vi "mlProject_testNetwork.vi"() -> ()   [LabVIEW 2016]
uses:
  <vilib>/Analysis/7linalg.llb/Real Matrix Exp.vi
  <vilib>/Analysis/Matrix/Numeric/Subtract/Subtract - RM,RM.vi
  <vilib>/Analysis/NI_AALBase.lvlib
  <vilib>/Analysis/Matrix/NI_Matrix.lvlib
panel:
  out "error":i32
  out "Coefficient error":sgl[][](array[numeric])
  in  "nesterov":bool=TRUE
  in  "lambda":sgl
  in  "gamma":sgl=0.9
  in  "milliseconds to wait":u32
  out "out desired":sgl[][](array[numeric])
  in  "validate":bool
  out "Error":sgl[](graph)
  in  "eta":sgl=0.0001
  in  "stop":bool
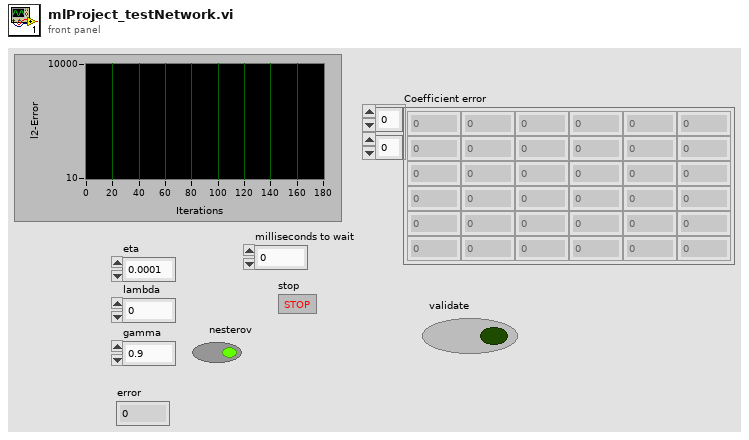
[diagram p1: front panel]
types:
  T1 = typedef "NI_Matrix.lvlib/RealMatrix.ctl" = dbl[][]
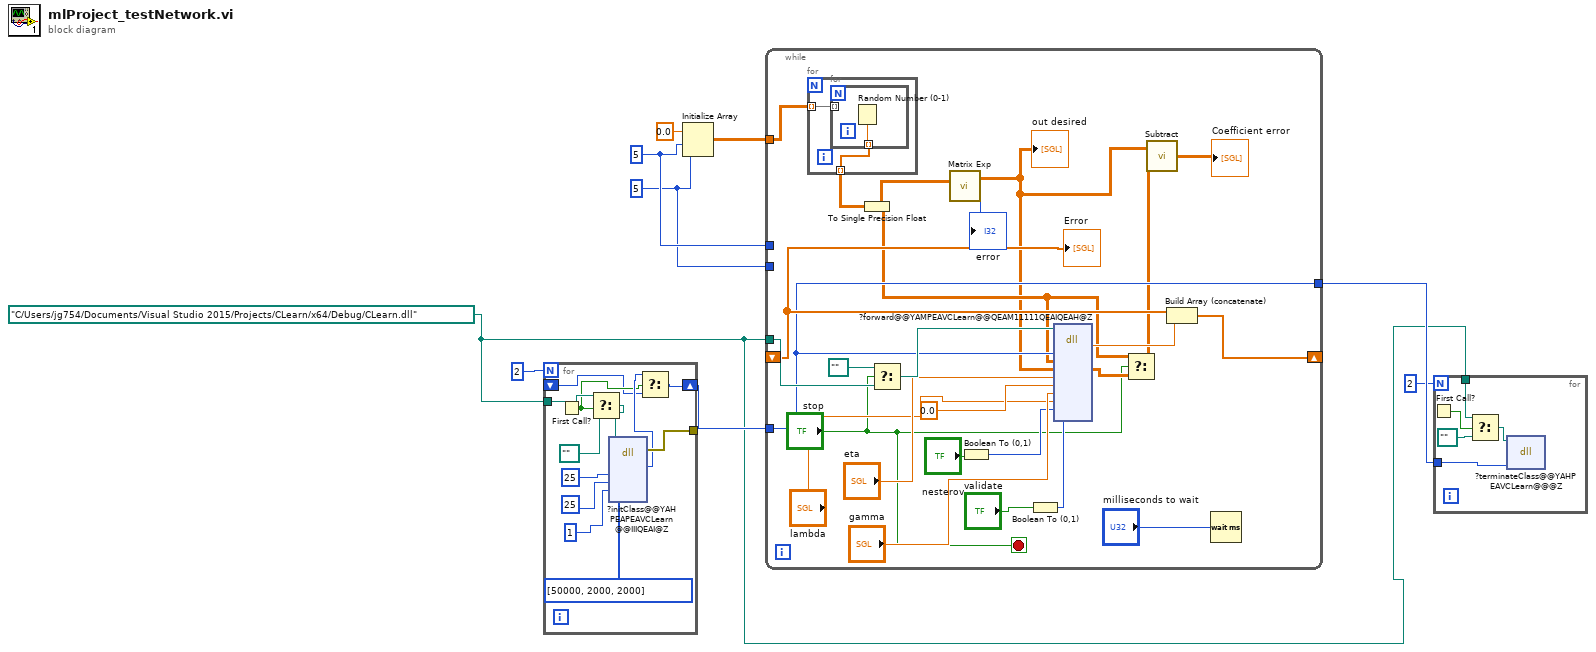
[diagram p0: block diagram]
diagram:
  w1 = 5 ("dimension size")
  w2 = 5 ("dimension size")
  w6 = path "C:/Users/jg754/Documents/Visual Studio 2015/Projects/CLearn/x64/Debug/CLearn.dll" ("path in")
  n1 = for {
    N: 2 -> [_]
    tunnel: w6 -> [w20]
    tunnel: [w21] -> _
    shift-right: [w17] -> w8
    shift-left: _ -> [w15]
    n2 = First Call?() -> (First Call?: T/F=w16:bool)
    n3 = Select(t=w20, s=w16, f=path "") -> (s? t:f=w19:path)
    n4 = dll-call lib="C:/Users/jg754/Documents/Visual Studio 2015/Projects/CLearn/x64/Debug/CLearn.dll" fn="?initClass@@YAHPEAPEAVCLearn@@IIIQEAI@Z"(path in=w19, "NIN"=u32 25, "NOUT"=u32 25, "NHIDDEN"=u32 1, "NNODES"=u32[] [50000, 2000, 2000]) -> (error out=w21:errorcluster, "ptr"=w18:i64)  [unwired: 8 in, 1 out]
    n5 = Select(t=w18, s=w16, f=w15) -> (s? t:f=w17:i64)
  }
  n6 = Initialize Array(0.0 ("element"), w2, w1) -> (w4:dbl[][])
  n7 = while {
    tunnel: w8 -> [w36]
    tunnel: w6 -> [w45]
    shift-right: [w41] -> _
    shift-left: _ -> [w40]
    tunnel: [w36] -> w7
    tunnel: w4 -> [w34]
    tunnel: w2 -> [_]
    tunnel: w1 -> [_]
    stop <- "stop" stop-if-true
    n8 = for {
      tunnel: w34 -> [w48] mode=indexing
      tunnel: [w47] -> w25 mode=indexing
      n9 = for {
        tunnel: w48 -> [_] mode=indexing
        tunnel: [w49] -> w47 mode=indexing
        n10 = Random Number (0-1)() -> (number: 0 to 1=w49:dbl)
      }
    }
    n11 = To Single Precision Float(number=w25) -> (single precision float=w24:sgl[][])
    n12 = Select(t=path "", s="stop", f=w45) -> (s? t:f=w44:path)
    n13 = call-poly <vilib>:"Matrix Exp.vi"("Input Matrix"=w24) -> ("error"=→"error":i32, "Matrix Exp"=w23:T1)  [unwired: 1 in]
    "out desired" <- w23
    n14 = Boolean To (0,1)(Boolean="nesterov") -> (0, 1=w29:i16)
    n15 = Boolean To (0,1)(Boolean="validate") -> (0, 1=w37:i16)
    n16 = dll-call lib="C:/Users/jg754/Documents/Visual Studio 2015/Projects/CLearn/x64/Debug/CLearn.dll" fn="?forward@@YAMPEAVCLearn@@QEAM11111QEAIQEAH@Z"(path in=w44, "ptr"=w36, "SLM"=w24, "image"=w23, "eta"="eta", "metaEta"=sgl 0.0, "gamma"="gamma", "lambda"="lambda", "nesterov"=w29, "validate"=w37) -> ("return type"=w42:sgl, "image"=w28:sgl[][])  [unwired: 10 in, 2 out]
    n17 = Select(t=w24, s="stop", f=w28) -> (s? t:f=w27:sgl[][])
    n18 = call-poly <vilib>:"Subtract.vi"("Real Matrix B"=w27, "Real Matrix A"=w23) -> ("A - B"=→"Coefficient error":T1)
    n19 = Build Array (concatenate)(w40, w42) -> (w41:sgl[])
    n20 = Wait (ms)(milliseconds to wait="milliseconds to wait") -> ()  [unwired: 1 out]
    "Error" <- w40
  }
  n21 = for {
    N: 2 -> [_]
    tunnel: w6 -> [w54]
    tunnel: w7 -> [w50]
    n22 = First Call?() -> (First Call?: T/F=w53:bool)
    n23 = Select(t=w54, s=w53, f=path "" ("t")) -> (s? t:f=w51:path)
    n24 = dll-call lib="C:/Users/jg754/Documents/Visual Studio 2015/Projects/CLearn/x64/Debug/CLearn.dll" fn="?terminateClass@@YAHPEAVCLearn@@@Z"(path in=w51, "ptr"=w50) -> ()  [unwired: 4 in, 2 out]
  }
